vi "Handle Error.vi"(8 "ErrorArrayIn":errorcluster[](array[cluster]), 11 "Message Queue":refnum<queue>) -> (0 "ErrorArrayOut":errorcluster[](array[cluster]))   [LabVIEW 2018, in "Message Queue.lvlib"]
uses:
  Message Queue.lvlib
  Message Cluster.ctl
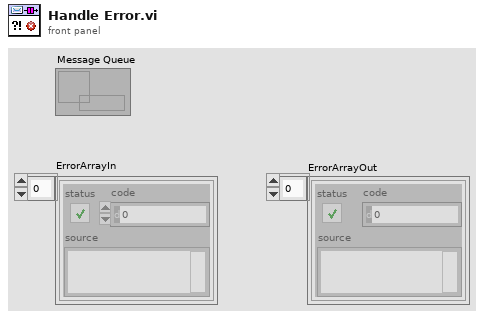
[diagram p1: front panel]
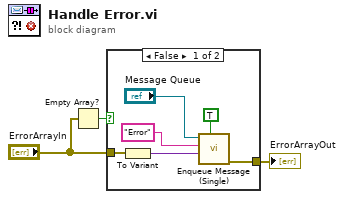
[diagram p0: block diagram]
diagram:
  n1 = Empty Array?(array="ErrorArrayIn") -> (empty?=w3:bool)
  n2 = case shown="False" w3 {
    tunnel: "ErrorArrayIn" -> [w8 w10]
    tunnel: [w5 w10] -> w1
    frame False {
      n3 = To Variant(anything=w8) -> (Variant=w9:variant)
      n4 = call "Enqueue Message (Single).vi"("Priority Message? (F)"=TRUE ("Priority (F)"), "Message Data"=w9, "Message"="Error", "Message Queue"="Message Queue") -> ("error out"=w5:errorcluster[])  [unwired: 6 in, 1 out]
    }
    frame True {
    }
  }
  "ErrorArrayOut" <- w1
